vi "Destroy.vi"(8 "error in (no error)":errorcluster, 11 "Result Model in":refnum<class "Result Model.lvclass">) -> (0 "error out":errorcluster)   [LabVIEW 2020, in "Result Model.lvclass"]
uses:
  Result Model/Result Model.lvclass
  Result Model/Result Model.lvclass/Result Model.ctl
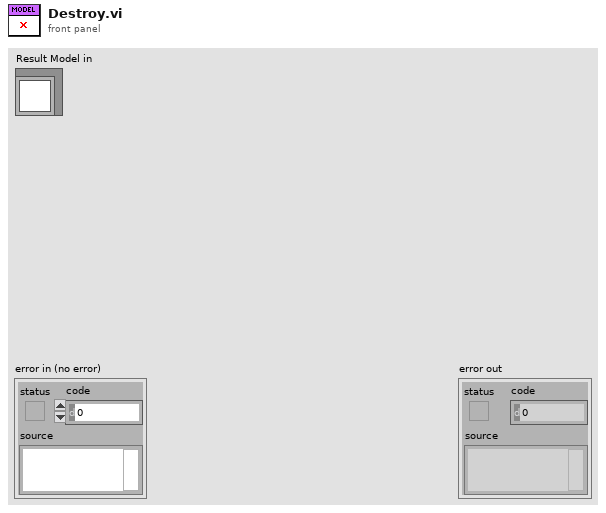
[diagram p1: front panel]
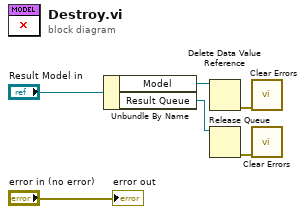
[diagram p0: block diagram]
diagram:
  n1 = Unbundle By Name("Result Model in") -> ("Model"=w3:refnum<data-value>, "Result Queue"=w2:refnum<queue>)
  n2 = Delete Data Value Reference(data value reference=w3) -> (error out=w5:errorcluster)  [unwired: 1 in, 1 out]
  n3 = Release Queue(queue=w2) -> (error out=w1:errorcluster)  [unwired: 2 in, 2 out]
  n4 = call <vilib>:"Clear Errors.vi"("error in (no error)"=w5) -> ()  [unwired: 5 in, 2 out]
  n5 = call <vilib>:"Clear Errors.vi"("error in (no error)"=w1) -> ()  [unwired: 5 in, 2 out]
  "error out" <- "error in (no error)"
